vi "LVClass_CorrectionDataManager UpdateInteractionMatrix.vi"(0 "CorrectionDataManager in":refnum<class "CorrectionDataManager.lvclass">, 5 "HasoSlopes push movement":refnum<class "HasoSlopes.lvclass">, 7 "HasoSlopes pull movement":refnum<class "HasoSlopes.lvclass">, 9 "Index of actuator":i32, 11 "error in (no error)":errorcluster) -> (4 "CorrectionDataManager out":refnum<class "CorrectionDataManager.lvclass">, 15 "error out":errorcluster)   [LabVIEW 2020, in "CorrectionDataManager.lvclass"]
uses:
  CorrectionDataManager.lvclass
  HasoSlopes.lvclass
  CorrectionDataManager.lvclass/CorrectionDataManager.ctl
  LVClass_HasoSlopes Read HasoSlopes _ property.vi
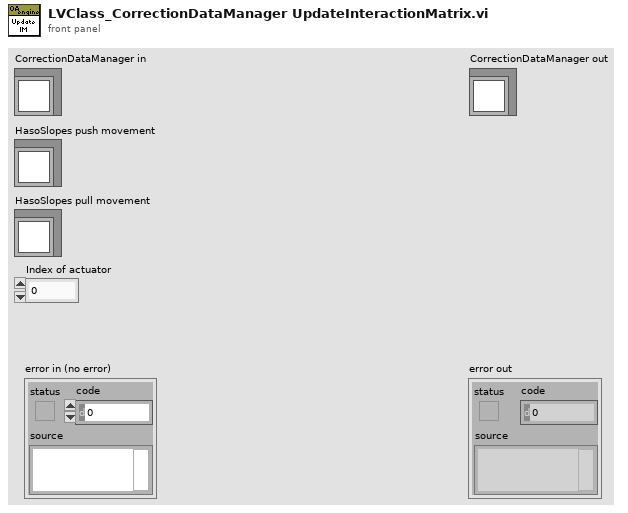
[diagram p1: front panel]
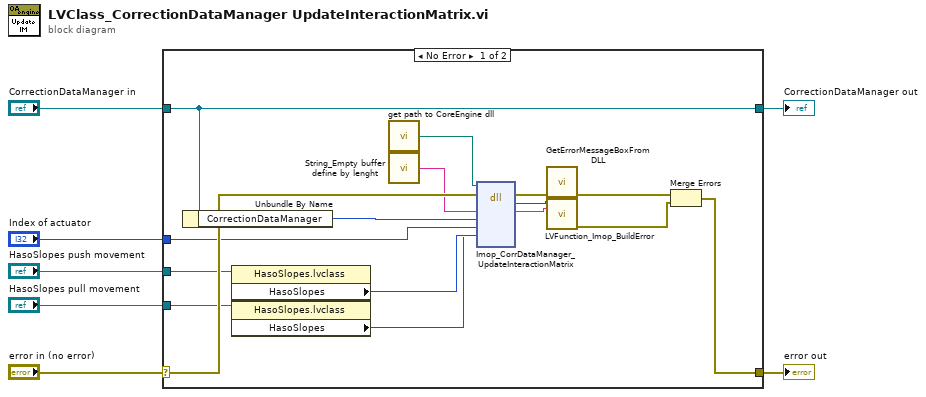
[diagram p0: block diagram]
diagram:
  n1 = case shown="No Error" "error in (no error)" {
    selector: "error in (no error)" -> [w20 w25]
    tunnel: [w21 w25] -> w6
    tunnel: [w9 w24] -> w4
    tunnel: "CorrectionDataManager in" -> [w9 w24]
    tunnel: "Index of actuator" -> [w14 _]
    tunnel: "HasoSlopes push movement" -> [w13 _]
    tunnel: "HasoSlopes pull movement" -> [w12 _]
    frame No Error {
      n2 = Unbundle By Name(w9) -> ("CorrectionDataManager"=w8:i32)
      n3 = property class="HasoSlopes.lvclass"(reference=w13) -> ("HasoSlopes"=w11:i32)  [unwired: 1 in, 2 out]
      n4 = property class="HasoSlopes.lvclass"(reference=w12) -> ("HasoSlopes"=w10:i32)  [unwired: 1 in, 2 out]
      n5 = call "get path to CoreEngine dll.vi"() -> ("path to c_interface_vc100.dll"=w18:path)  [unwired: 12 in, 3 out]
      n6 = call "String_Empty buffer define by lenght.vi"() -> ("Empty buffer"=w15:string)  [unwired: 1 in]
      n7 = dll-call lib="D:/FLE/0.Code/CoreEngine4_Suite/LV2011_interface/DLLs/c_interface_vc100.dll" fn="Imop_CorrDataManager_UpdateInteractionMatrix"(path in=w18, error in=w20, "Message"=w15, "Correction Data Manager"=w8, "Index of actuator"=w14, "HasoSlopes push"=w11, "Haso Slopes pull"=w10) -> (error out=w19:errorcluster, "return type"=w17:i32, "Message"=w16:string)  [unwired: 5 in, 1 out]
      n8 = call "GetErrorMessageBoxFromDLL.vi"("error IN"=w19) -> ("error OUT"=w23:errorcluster)  [unwired: 10 in]
      n9 = call "LVFunction_Imop_BuildError.vi"("code"=w17, "String to Prepend to source (\"\")"=w16) -> ("error out"=w22:errorcluster)  [unwired: 13 in]
      n10 = Merge Errors(w23, w22) -> (w21:errorcluster)
    }
    frame Error {
    }
  }
  "error out" <- w6
  "CorrectionDataManager out" <- w4
